vi "Grid Measurements Example - Topo & GridSpectr_DriftCorrection.vi"(6 "Internal use":string, 7 "Grid param":T1 {"height (m)" format="%#_6p"; "width (m)" format="%#_6p"; "center Y (m)" format="%#_6p"; "center X (m)" format="%#_6p"}, 8 "Error in (no error)":errorcluster, 9 "Points Y/Index Y":i32, 10 "Points X/Index X":i32, 11 "Method":enum16{"init", "run", "end"}(ring)=enum."end") -> (0 "Error out":errorcluster)   [LabVIEW 2014]
doc: "Example of a measurement VI to be used in the \"Experiments on a Grid\" tool as external VI.\n\nThis example measure the topography and spectroscopy data. The spectroscopy measurements are taken on a subgrid. The data are saved to a sxm and a binary file.\n\n- Nanonis Programming Interface -"
uses:
  <vilib>/Analysis/2dsp.llb/2D Cross Correlation (DBL).vi
  <userlib>/Nanonis Prog Interface V5/Nanonis Prog Interface.lvlib
  <vilib>/Analysis/NI_AALPro.lvlib
panel:
  in  "File name":string
  in  "STS Current":dbl format="%#_6p"
  in  "Imaging Current":dbl format="%#_6p"
  in  "zdrift \nDuration (s)":dbl
  in  "Correct z drift":bool
  out "Status":string="init"
  in  "Drift correction Pixels":i32=128 caption="Pixels for drift correction"
  out "Y Offset":dbl
  out "X Offset":dbl
  out "Points taken":dbl=1.0
  in  "Drift Correction":i32=128
  in  "Y subgrid spacing":u16=1
  in  "X subgrid spacing":u16=1
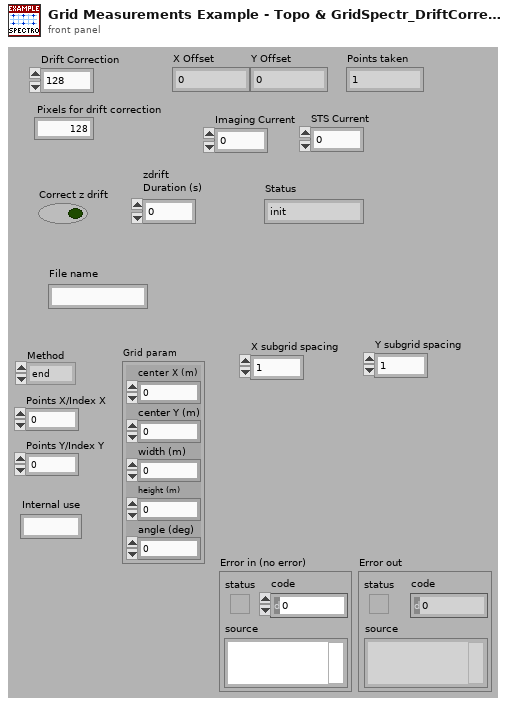
[diagram p1: front panel]
types:
  T1 = cluster{"center X (m)":sgl, "center Y (m)":sgl, "width (m)":sgl, "height (m)":sgl, "angle (deg)":sgl}
  T2 = enum16{"open", "replace", "create", "open or create", "replace or create", "replace or create with confirmation"}
  T3 = cluster{"center X":sgl, "center Y":sgl, "angle":sgl, "width":sgl, "height":sgl, "# pixels":i32, "# lines":i32}
  T4 = cluster{"Name":string, "Calibration":sgl, "Offset":sgl, "Channel index":i32}[]
  T5 = cluster{"up/down":bool, "time/line":sgl, "start time":timestamp, "end time":timestamp}
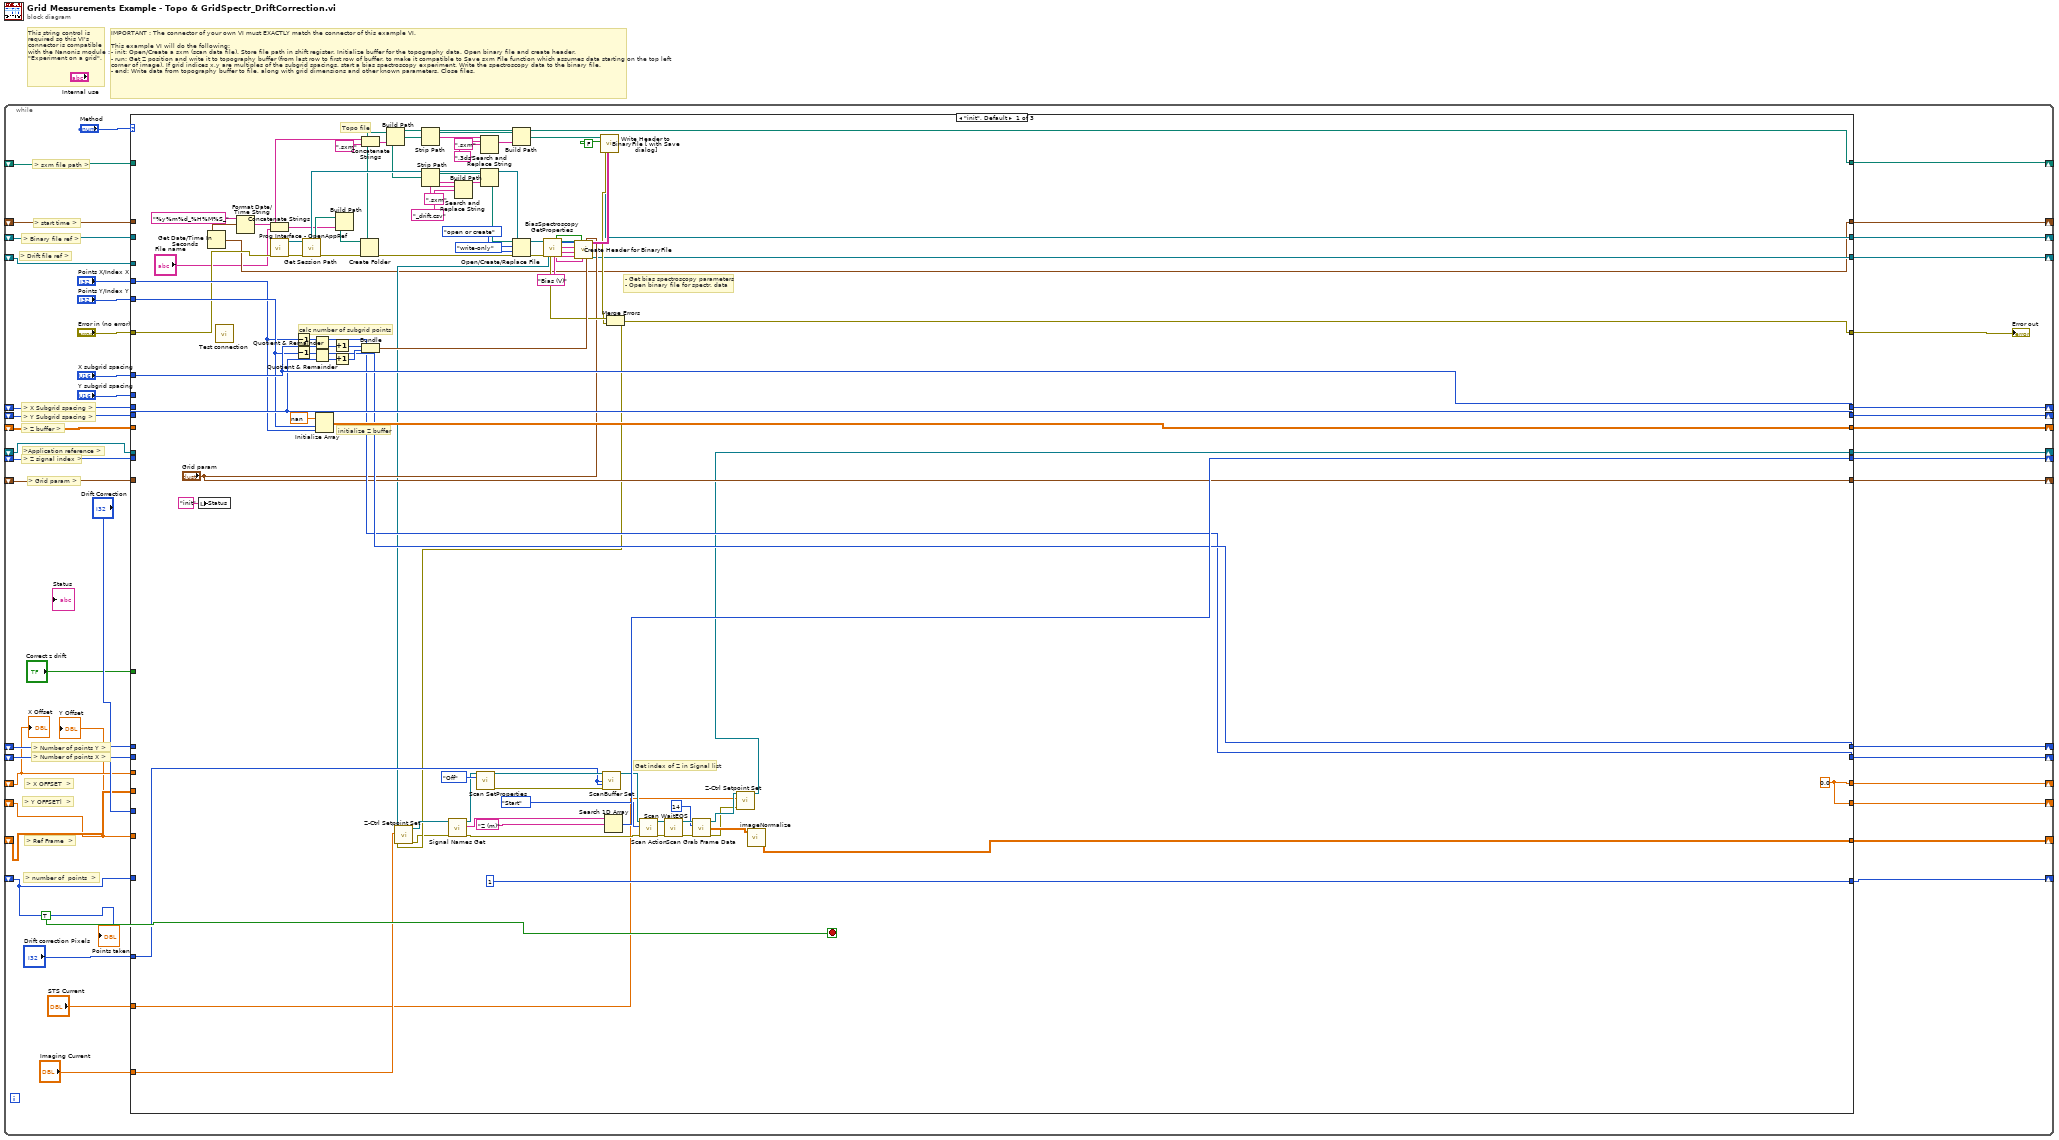
[diagram p0: block diagram]
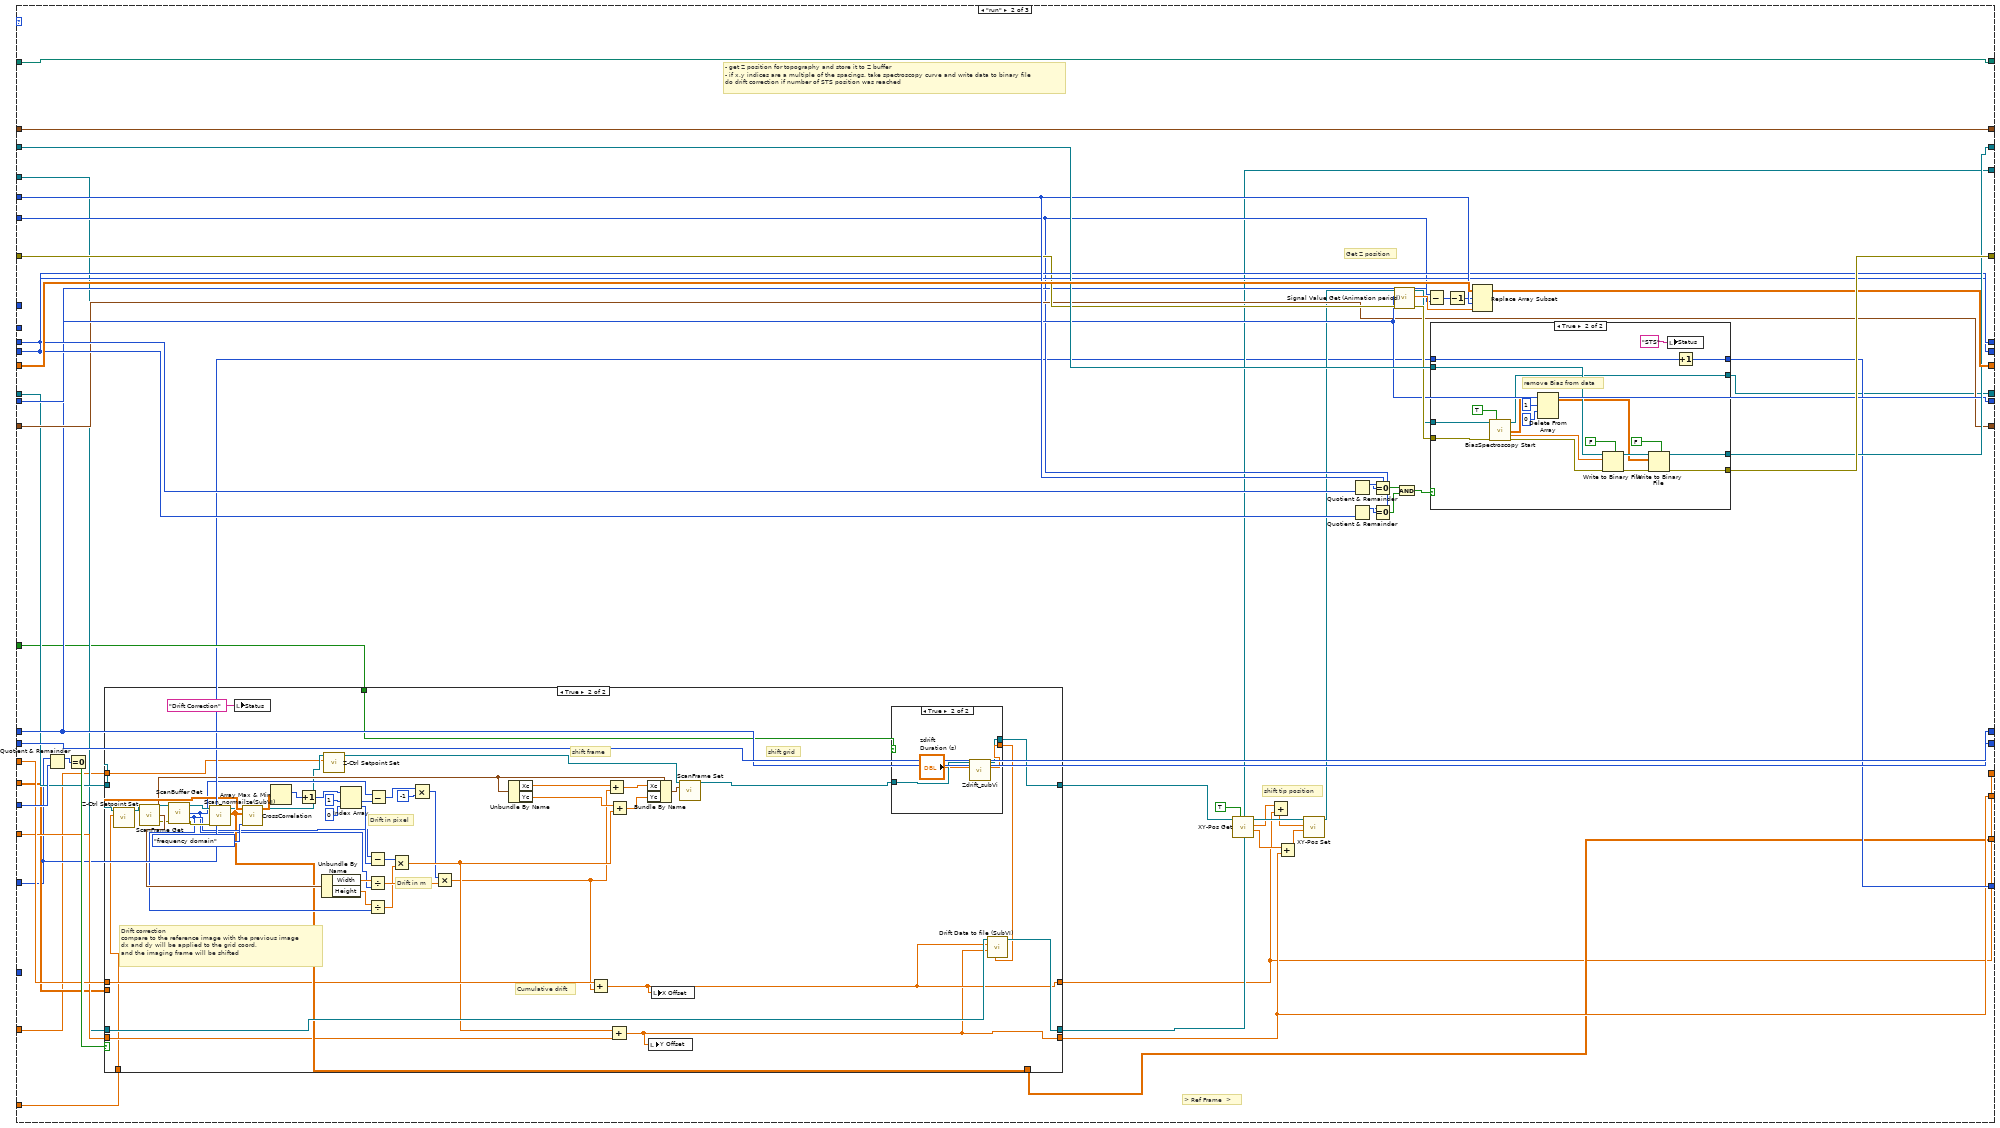
[diagram p2: hidden frame]
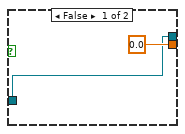
[diagram p4: hidden frame]
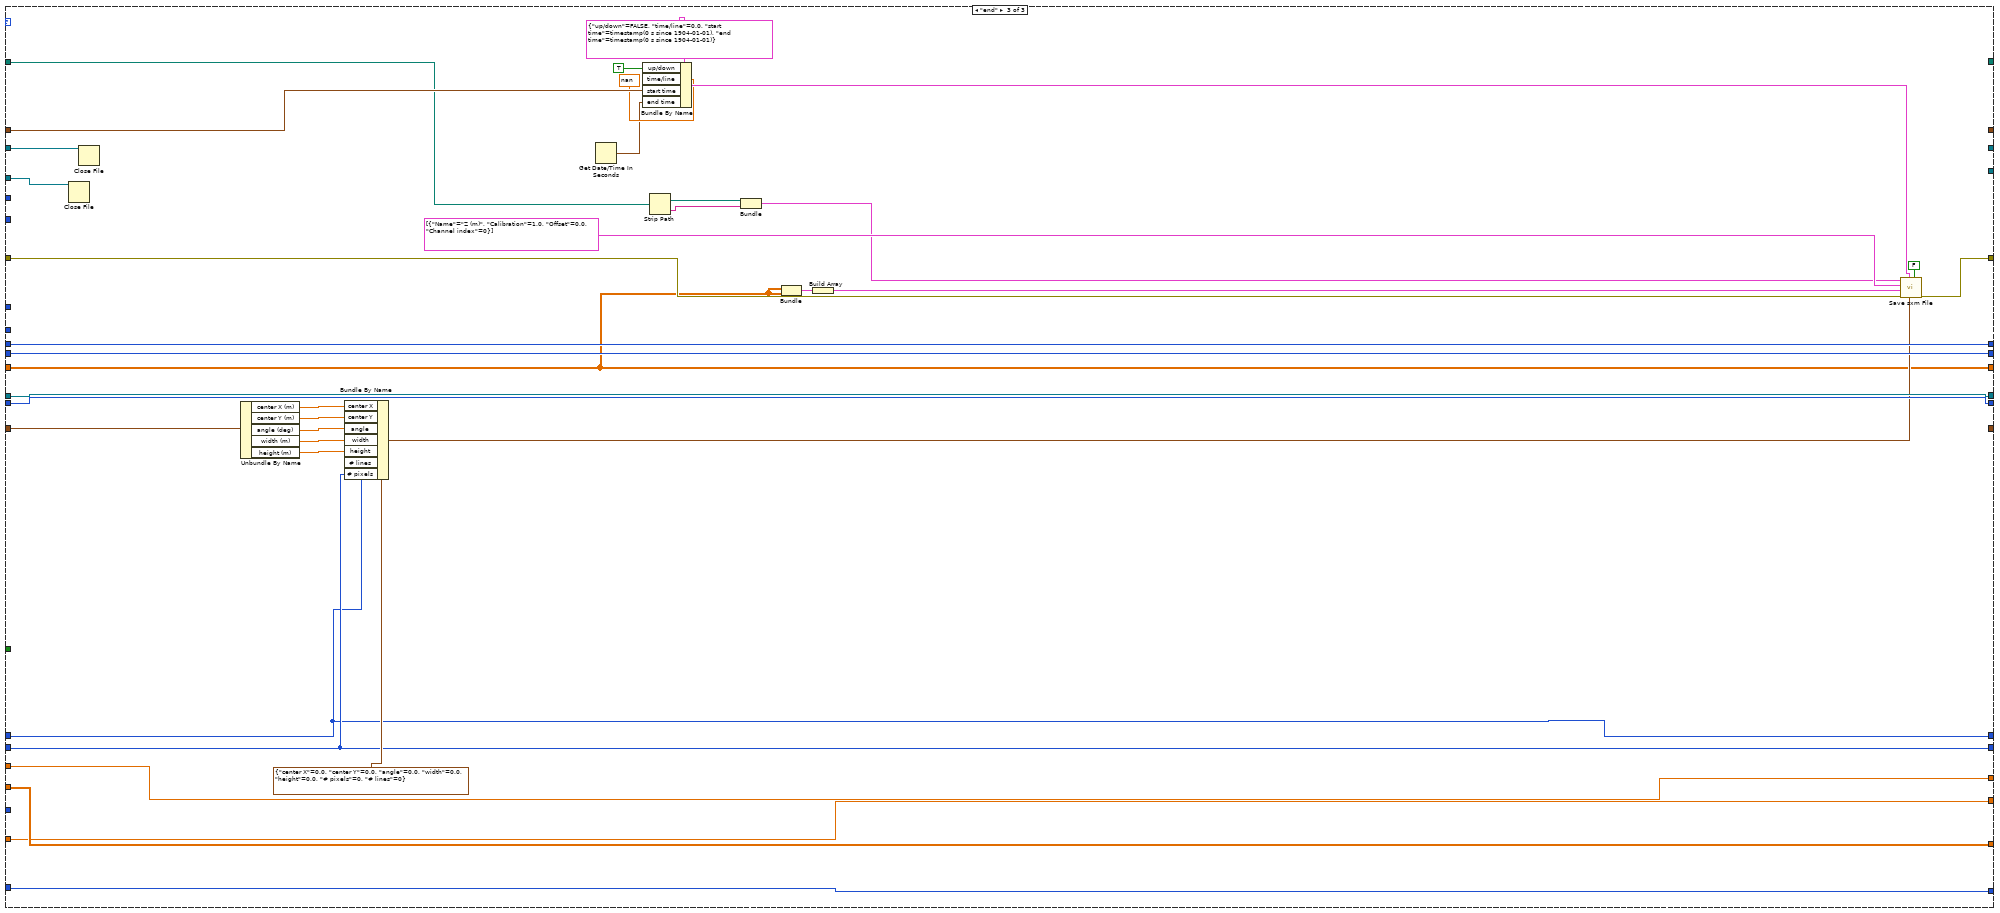
[diagram p6: hidden frame]
diagram:
  # "This string control is required so this VI's connector is compatible with the Nanonis module : \"Experiment on a grid\"."
  # "IMPORTANT : The connector of your own VI must EXACTLY match the connector of this example VI.\n\nThis example VI will do the following:\n- init: Open/Create a sxm (scan data file). Store file path in shift register. Initialize buffer for the topography data. Open binary file and create header.\n- run: Get Z position and write it to topography buffer (from last row to first row of buffer, to make it compatible to Save sxm File function which assumes data starting on the top left corner of image). If grid indices x,y are multiples of the subgrid spacings, start a bias spectroscopy experiment. Write the spectroscopy data to the binary file.\n- end: Write data from topography buffer to file, along with grid dimensions and other known parameters. Close files."
  n1 = while {
    shift-right: [w20] -> _
    shift-left: _ -> [w43]
    shift-right: [w38] -> _
    shift-left: _ -> [w37]
    shift-right: [w35] -> _
    shift-left: _ -> [w36]
    shift-right: [w34] -> _
    shift-left: _ -> [w33]
    shift-right: [w27] -> _
    shift-left: _ -> [w29]
    shift-right: [w28] -> _
    shift-left: _ -> [w30]
    shift-right: [w26] -> _
    shift-left: _ -> [w25]
    shift-right: [w24] -> _
    shift-left: _ -> [w23]
    shift-right: [w22] -> _
    shift-left: _ -> [w21]
    shift-right: [w19] -> _
    shift-left: _ -> [w18]
    shift-right: [w17] -> _
    shift-left: _ -> [w16]
    shift-right: [w15] -> _
    shift-left: _ -> [w8]
    shift-right: [w14] -> _
    shift-left: _ -> [w7]
    shift-right: [w13] -> _
    shift-left: _ -> [w10]
    shift-right: [w12] -> _
    shift-left: _ -> [w9]
    shift-right: [w5] -> _
    shift-left: _ -> [w4]
    stop <- TRUE stop-if-true
    # "> Drift file ref >"
    # "> number of  points  >"
    # "> Ref Frame  >"
    # "> Y OFFSETl  >"
    # "> X OFFSET  >"
    # "> Number of points X >"
    # "> Number of points Y >"
    # "> Grid param >"
    # "> start time >"
    # ">Application reference >"
    # "> Y Subgrid spacing >"
    # "> X Subgrid spacing >"
    # "> Z signal index >"
    # "> Binary file ref >"
    # "> Z buffer >"
    # "> sxm file path >"
    n2 = case shown="\"init\", Default" "Method" {
      tunnel: [w52 w185 _] -> w20
      tunnel: w43 -> [_ w185 w297]
      tunnel: "Error in (no error)" -> [w59 w171 w290]
      tunnel: [w69 w184 w289] -> w41
      tunnel: "Points X/Index X" -> [w108 w179 _]
      tunnel: "Points Y/Index Y" -> [w109 w163 _]
      tunnel: [w133 w182 w278] -> w38
      tunnel: w37 -> [_ w183 w278]
      tunnel: w36 -> [_ w181 w306]
      tunnel: [w124 w180 _] -> w35
      tunnel: [w122 w169 w307] -> w34
      tunnel: w33 -> [_ w169 w307]
      tunnel: "X subgrid spacing" -> [w121 _ _]
      tunnel: "Y subgrid spacing" -> [w120 _ _]
      tunnel: w30 -> [_ w173 w305]
      tunnel: w29 -> [_ w172 w304]
      tunnel: [w121 w173 w305] -> w28
      tunnel: [w120 w172 w304] -> w27
      tunnel: [w66 w154 w303] -> w26
      tunnel: w25 -> [_ w153 w303]
      tunnel: ["Grid param" w166 _] -> w24
      tunnel: w23 -> [_ w166 w288]
      tunnel: [w49 w167 _] -> w22
      tunnel: w21 -> [_ w167 w298]
      tunnel: [w109 w164 w279] -> w19
      tunnel: w18 -> [_ w164 w279]
      tunnel: [w108 w165 w280] -> w17
      tunnel: w16 -> [_ w165 w280]
      tunnel: [w98 w136 w277] -> w15
      tunnel: [w98 w143 w274] -> w14
      tunnel: [w74 w141 w276] -> w13
      tunnel: [1 w160 w275] -> w12
      tunnel: w9 -> [_ w137 w275]
      tunnel: "Drift Correction" -> [_ w158 _]
      tunnel: w10 -> [_ w142 w276]
      tunnel: w8 -> [_ w156 w277]
      tunnel: w7 -> [_ w155 w274]
      tunnel: "Drift correction Pixels" -> [w94 _ _]
      tunnel: [w87 w139 _] -> w5
      tunnel: w4 -> [_ w140 w271]
      tunnel: "Correct z drift" -> [_ w138 _]
      tunnel: "Imaging Current" -> [w70 w135 _]
      tunnel: "STS Current" -> [w64 w134 _]
      frame "init", Default {
        w98 = 0.0
        # "Topo file"
        # "- Get bias spectroscopy parameters\n- Open binary file for spectr. data"
        # "initialize Z buffer"
        # "calc number of subgrid points"
        # "Get index of Z in Signal list"
        n3 = local write "Status"("init" ("Status")) -> ()
        n4 = Get Date/Time In Seconds() -> (seconds since 1Jan1904=w49:timestamp)
        n5 = call <userlib>:"Test connection.vi"() -> ()  [unwired: 1 in]
        n6 = Format Date/Time String(time format string (%c)="%y%m%d_%H%M%S_", seconds (now)=w49) -> (date/time string=w48:string)  [unwired: 1 in]
        n7 = Concatenate Strings(w48, "File name") -> (w50:string)
        n8 = call <userlib>:"Prog Interface - OpenAppRef.vi"("Error in (no error)"=w59) -> ("Error out"=w61:errorcluster, "Application reference"=w63:refnum<vi>)  [unwired: 5 in]
        n9 = Decrement(x=w108) -> (x-1=w119:i32)
        n10 = Decrement(x=w109) -> (x-1=w118:i32)
        n11 = call <userlib>:"Get Session Path.vi"("error in (no error)"=w61, "Application ref in"=w63) -> ("error out"=w57:errorcluster, "Session path"=w60:path, "Application ref out"=w62:refnum<vi>)  [unwired: 7 in]
        n12 = Quotient & Remainder(x=w119, y=w121) -> (floor(x/y)=w117:i32)  [unwired: 1 out]
        n13 = Quotient & Remainder(x=w118, y=w120) -> (floor(x/y)=w116:i32)  [unwired: 1 out]
        n14 = Initialize Array(sgl nan ("element"), w109, w108) -> (w133:sgl[][])
        n15 = Increment(x=w117) -> (x+1=w115:i32)
        n16 = Increment(x=w116) -> (x+1=w114:i32)
        n17 = Build Path(base path=w60, name or relative path=w50) -> (appended path=w56:path)
        n18 = Create Folder(path (use dialog)=w56, error in=w57) -> (created path=w54:path, error out=w51:errorcluster)  [unwired: 1 in, 1 out]
        n19 = Concatenate Strings(w50, ".sxm" ("pattern")) -> (w53:string)
        n20 = Bundle(w115, w114) -> (w128:cluster{i32, i32})  [unwired: 1 in]
        n21 = Build Path(base path=w54, name or relative path=w53) -> (appended path=w52:path)
        n22 = Strip Path(path=w52) -> (stripped path=w80:path, name=w79:string)
        n23 = Strip Path(path=w52) -> (stripped path=w89:path, name=w85:string)
        n24 = Search and Replace String(input string=w85, search string=".sxm", replace string="_drift.csv" ("replace string (\"\")")) -> (result string=w86:string)  [unwired: 5 in, 3 out]
        n25 = Search and Replace String(input string=w79, search string=".sxm", replace string=".3ds" ("replace string (\"\")")) -> (result string=w81:string)  [unwired: 5 in, 3 out]
        n26 = Build Path(base path=w89, name or relative path=w86) -> (appended path=w88:path)
        n27 = Build Path(base path=w80, name or relative path=w81) -> (appended path=w76:path)
        n28 = Open/Create/Replace File(file path (use dialog)=w88, error in=w51, operation (0:open)=T2."open or create", access (0:read/write)=enum16{"read/write", "read-only", "write-only"}."write-only") -> (refnum out=w87:refnum<file>, error out=w58:errorcluster)  [unwired: 2 in, 1 out]
        n29 = call <userlib>:"BiasSpectroscopy GetProperties.vi"("Application ref in"=w62, "Error in (no error)"=w58) -> ("Backward sweep"=w129:bool, "Application ref out"=w72:refnum<vi>, "Number of points"=w111:i32, "Channels"=w110:string[], "Parameters"=w127:string[], "Fixed parameters"=w113:string[], "Error out"=w126:errorcluster)  [unwired: 5 in, 2 out]
        n30 = call <userlib>:"Create Header for BinaryFile.vi"("Grid points"=w128, "Grid param"="Grid param", "Fixed parameters"=w113, "Backward sweep"=w129, "Sweep signal"="Bias (V)" ("Sweep Signal"), "Parameters"=w127, "Channels"=w110, "Points per sweep"=w111) -> ("Header (fixed attributes)"=w131:string[][])  [unwired: 3 in]
        n31 = call <userlib>:"Write Header to BinaryFile [ with Save dialog].vi"("Fixed Attributes"=w131, "Show Dialog? (T)"=FALSE, "Filename"=w76) -> ("Error out"=w125:errorcluster, "File ref"=w124:refnum<file>)  [unwired: 5 in, 2 out]
        n32 = Merge Errors(w126, w125) -> (w69:errorcluster)
        n33 = call <userlib>:"Z-Ctrl Setpoint Set.vi"("error in (no error)"=w69, "Z Controller setpoint"=w70, "Application ref in"=w72) -> ("error out"=w68:errorcluster, "Application ref out"=w71:refnum<vi>)  [unwired: 7 in]
        n34 = call <userlib>:"Signal Names Get.vi"("error in (no error)"=w68, "Application ref in"=w71) -> ("error out"=w99:errorcluster, "Signals Names"=w112:string[], "Application ref out"=w93:refnum<vi>)  [unwired: 5 in]
        n35 = call <userlib>:"Scan SetProperties.vi"("Application ref in"=w93, "Continuous scan"=enum16{"No change", "On", "Off"}."Off") -> ("Application ref out"=w96:refnum<vi>, "Error out"=w95:errorcluster)  [unwired: 12 in]
        n36 = call <userlib>:"ScanBuffer Set.vi"("Application ref in"=w96, "Pixels"=w94, "Lines"=w94, "error in (no error)"=w95) -> ("Application ref out"=w92:refnum<vi>)  [unwired: 10 in, 1 out]
        n37 = Search 1D Array(1D array=w112, element="Z (m)") -> (index of element=w122:i32)  [unwired: 1 in]
        n38 = call <userlib>:"Scan Action.vi"("error in (no error)"=w99, "Scan action (Start)"=enum16{"Start", "Stop", "Pause", "Resume"}."Start", "Application ref in"=w92) -> ("error out"=w106:errorcluster, "Application ref out"=w105:refnum<vi>)  [unwired: 6 in]
        n39 = call <userlib>:"Scan WaitEOS.vi"("error in (no error)"=w106, "Application ref in"=w105) -> ("error out"=w103:errorcluster, "Application ref out"=w104:refnum<vi>)  [unwired: 5 in, 2 out]
        n40 = call <userlib>:"Scan Grab Frame Data.vi"("Application ref in"=w104, "Channel index (0-23)"=u8 14, "error in (no error)"=w103) -> ("Application ref out"=w67:refnum<vi>, "Scan frame data"=w73:sgl[][], "error out"=w65:errorcluster)  [unwired: 8 in, 2 out]
        n41 = call <userlib>:"Z-Ctrl Setpoint Set.vi"("error in (no error)"=w65, "Z Controller setpoint"=w64, "Application ref in"=w67) -> ("Application ref out"=w66:refnum<vi>)  [unwired: 7 in, 1 out]
        n42 = call "imageNormalize.vi"("Data"=w73) -> ("Array"=w74:dbl[][])  [unwired: 10 in]
      }
      frame "run" {
        # "> Ref Frame  >"
        # "shift tip position"
        # "Get Z position"
        # "- get Z position for topography and store it to Z buffer\n- if x,y indices are a multiple of the spacings, take spectroscopy curve and write data to binary file\ndo drift correction if number of STS position was reached"
        n43 = Quotient & Remainder(x=w137, y=w158) -> (x-y*floor(x/y)=w159:i32)  [unwired: 1 out]
        n44 = Equal To 0?(x=w159) -> (x = 0?=w157:bool)
        n45 = case shown="True" w157 {
          tunnel: w153 -> [w190 w201]
          tunnel: [w190 w212] -> w152
          tunnel: w142 -> [w187 w218]
          tunnel: [w189 w205] -> w136
          tunnel: [w188 w204] -> w143
          tunnel: w156 -> [w189 w209]
          tunnel: w155 -> [w188 w210]
          tunnel: [w187 w211] -> w141
          tunnel: w140 -> [w186 w217]
          tunnel: [w186 w216] -> w139
          tunnel: w138 -> [_ w208]
          tunnel: w135 -> [_ w199]
          tunnel: w134 -> [_ w196]
          frame False {
          }
          frame True {
            # "shift grid"
            # "Cumulative drift"
            # "shift frame"
            # "Drift in m"
            # "Drift in pixel"
            # "Drift correction \ncompare to the reference image with the previous image \ndx and dy will be applied to the grid coord, \nand the imaging frame will be shifted"
            n46 = call <userlib>:"Z-Ctrl Setpoint Set.vi"("Z Controller setpoint"=w199, "Application ref in"=w201) -> ("Application ref out"=w200:refnum<vi>)  [unwired: 8 in, 1 out]
            n47 = call <userlib>:"ScanFrame Get.vi"("Application ref in"=w200) -> ("Application ref out"=w234:refnum<vi>, "Center coordinates (m)"=w206:cluster{"Xc":sgl, "Yc":sgl}, "Size (m)"=w232:cluster{"Width":sgl, "Height":sgl}, "error out"=w231:errorcluster)  [unwired: 10 in, 1 out]
            n48 = call <userlib>:"ScanBuffer Get.vi"("Application ref in"=w234, "error in (no error)"=w231) -> ("Application ref out"=w230:refnum<vi>, "Pixels/line"=w207:i32, "Lines"=w220:i32, "error out"=w229:errorcluster)  [unwired: 9 in, 1 out]
            n49 = call "Scan_normailze(SubVI).vi"("error in (no error)"=w229, "Application in"=w230) -> ("Array"=w211:dbl[][], "Application out"=w198:refnum<vi>)  [unwired: 7 in, 1 out]
            n50 = local write "Status"("Drift Correction" ("Status")) -> ()
            n51 = call-poly <vilib>:"CrossCorrelation.vi"("algorithm"=enum32{"direct", "frequency domain"}."frequency domain", "Y"=w211, "X"=w218) -> ("Rxy"=w237:dbl[][])  [unwired: 7 in, 1 out]
            n52 = Array Max & Min(array=w237) -> (max index (indices)=w192:i32[])  [unwired: 3 out]
            n53 = Increment(x=w192) -> (x+1=w191:i32[])
            n54 = Unbundle By Name(w232) -> ("Width"=w228:sgl, "Height"=w233:sgl)
            n55 = call <userlib>:"Z-Ctrl Setpoint Set.vi"("Z Controller setpoint"=w196, "Application ref in"=w198) -> ("Application ref out"=w197:refnum<vi>)  [unwired: 8 in, 1 out]
            n56 = Index Array(array=w191, index #1=1 ("index"), index #2=0 ("index")) -> (element #1=w236:i32, element #2=w235:i32)
            n57 = Subtract(x=w220, y=w235) -> (x-y=w213:i32)
            n58 = Divide(x=w228, y=w207) -> (x/y=w227:sgl)
            n59 = Divide(x=w233, y=w220) -> (x/y=w226:sgl)
            n60 = Subtract(x=w207, y=w236) -> (x-y=w214:i32)
            n61 = Multiply(x=w213, y=w226) -> (x*y=w203:sgl)
            n62 = Multiply(x=w214, y=-1) -> (x*y=w194:i32)
            n63 = Multiply(x=w194, y=w227) -> (x*y=w202:sgl)
            n64 = Unbundle By Name(w206) -> ("Xc"=w224:sgl, "Yc"=w222:sgl)
            n65 = Add(x=w209, y=w202) -> (x+y=w205:dbl)
            n66 = Add(x=w224, y=w202) -> (x+y=w223:sgl)
            n67 = Add(x=w203, y=w210) -> (x+y=w204:dbl)
            n68 = Add(x=w222, y=w203) -> (x+y=w221:sgl)
            n69 = Bundle By Name(cluster=w206, "Xc"=w223, "Yc"=w221) -> (w225:cluster{"Xc":sgl, "Yc":sgl})
            n70 = local write "Y Offset"(w204) -> ()
            n71 = local write "X Offset"(w205) -> ()
            n72 = call <userlib>:"ScanFrame Set.vi"("Application ref in"=w197, "Center coordinates (m)"=w225) -> ("Application ref out"=w195:refnum<vi>)  [unwired: 12 in, 1 out]
            n73 = case shown="True" w208 {
              tunnel: [0.0 ("z drift") w246] -> w215
              tunnel: w195 -> [w241 w245]
              tunnel: [w241 w244] -> w212
              frame False {
              }
              frame True {
                n74 = call "Zdrift_subVi.vi"("Duration"="zdrift \nDuration (s)", "Application in"=w245) -> ("z drift"=w246:dbl, "Application out"=w244:refnum<vi>)  [unwired: 7 in, 1 out]
              }
            }
            n75 = call "Drift Data to file (SubVI).vi"("z drift"=w215, "y Drift"=w204, "X drift"=w205, "Byte Stream File in"=w217) -> ("Byte Stream File out"=w216:refnum<file>)  [unwired: 7 in]
          }
        }
        n76 = call <userlib>:"XY-Pos Get.vi"("Wait for newest data (F=False)"=TRUE, "Application ref in"=w152) -> ("Y (m)"=w147:sgl, "X (m)"=w148:sgl, "Application ref out"=w149:refnum<vi>)  [unwired: 5 in, 1 out]
        n77 = Add(x=w148, y=w136) -> (x+y=w146:dbl)
        n78 = Add(x=w147, y=w143) -> (x+y=w145:dbl)
        n79 = call <userlib>:"XY-Pos Set.vi"("Y (m)"=w145, "X (m)"=w146, "Application ref in"=w149) -> ("Application ref out"=w150:refnum<vi>)  [unwired: 5 in, 1 out]
        n80 = Quotient & Remainder(x=w179, y=w173) -> (x-y*floor(x/y)=w178:i32)  [unwired: 1 out]
        n81 = Quotient & Remainder(x=w163, y=w172) -> (x-y*floor(x/y)=w177:i32)  [unwired: 1 out]
        n82 = Equal To 0?(x=w178) -> (x = 0?=w176:bool)
        n83 = Equal To 0?(x=w177) -> (x = 0?=w175:bool)
        n84 = call <userlib>:"Signal Value Get (Animation period).vi"("error in (no error)"=w171, "Signal index (0-47)"=w169, "Application ref in"=w150) -> ("error out"=w170:errorcluster, "Signal value"=w168:sgl, "Application ref out"=w151:refnum<vi>)  [unwired: 5 in]
        n85 = And(x=w176, y=w175) -> (x .and. y?=w174:bool)
        n86 = Subtract(x=w164, y=w163) -> (x-y=w162:i32)
        n87 = case shown="True" w174 {
          tunnel: [w249 w254] -> w184
          tunnel: w181 -> [w250 w270]
          tunnel: [w250 w268] -> w180
          tunnel: w170 -> [w249 w267]
          tunnel: w151 -> [w248 w259]
          tunnel: [w248 w258] -> w154
          tunnel: [w247 w252] -> w160
          tunnel: w137 -> [w247 w253]
          frame False {
            # "Point indices aren't multiple of subgrid spacing\n=> no spectroscopy at this point"
          }
          frame True {
            # "remove Bias from data"
            n88 = call <userlib>:"BiasSpectroscopy Start.vi"("Application ref in"=w259, "Get data (F)"=TRUE ("Get Data (F)"), "Error in (no error)"=w267) -> ("Application ref out"=w258:refnum<vi>, "Data"=w266:sgl[][], "Parameters"=w265:sgl[], "Error out"=w256:errorcluster)  [unwired: 8 in, 1 out]
            n89 = Delete From Array(array=w266, length=1, index (row)=0 ("index")) -> (array with subset deleted=w264:sgl[][])  [unwired: 1 in, 1 out]
            n90 = Write to Binary File(file (use dialog)=w270, data=w265, error in=w256, 5:FALSE ("prepend array or string size? (T)")) -> (refnum out=w269:refnum<file>, error out=w255:errorcluster)  [unwired: 2 in, 1 out]
            n91 = Write to Binary File(file (use dialog)=w269, data=w264, error in=w255, 5:FALSE ("prepend array or string size? (T)")) -> (refnum out=w268:refnum<file>, error out=w254:errorcluster)  [unwired: 2 in, 1 out]
            n92 = local write "Status"("STS" ("Status")) -> ()
            n93 = Increment(x=w253) -> (x+1=w252:i32)
          }
        }
        n94 = Decrement(x=w162) -> (x-1=w161:i32)
        n95 = Replace Array Subset(array=w183, new element=w168, index (row)=w161, index (col)=w179) -> (w182:sgl[][])
      }
      frame "end" {
        n96 = Close File(refnum=w271) -> ()  [unwired: 1 in, 2 out]
        n97 = Close File(refnum=w306) -> ()  [unwired: 1 in, 2 out]
        n98 = Unbundle By Name(w288) -> ("center X (m)"=w286:sgl, "center Y (m)"=w285:sgl, "angle (deg)"=w284:sgl, "width (m)"=w283:sgl, "height (m)"=w282:sgl)
        n99 = Bundle By Name(cluster=T3 {"center X"=0.0, "center Y"=0.0, "angle"=0.0, "width"=0.0, "height"=0.0, "# pixels"=0, "# lines"=0} ("Scanfield"), "center X"=w286, "center Y"=w285, "angle"=w284, "width"=w283, "height"=w282, "# lines"=w279, "# pixels"=w280) -> (w281:T3)
        n100 = Get Date/Time In Seconds() -> (seconds since 1Jan1904=w273:timestamp)
        n101 = Bundle By Name(cluster=T5 {"up/down"=FALSE, "time/line"=0.0, "start time"=timestamp(0 s since 1904-01-01), "end time"=timestamp(0 s since 1904-01-01)} ("Scan param"), "up/down"=TRUE, "time/line"=sgl nan ("input 7"), "start time"=w298, "end time"=w273) -> (w296:T5)
        n102 = Strip Path(path=w297) -> (stripped path=w293:path, name=w292:string)
        n103 = Bundle("stripped path"=w293, "name"=w292) -> (w291:cluster{"stripped path":path, "name":string})  [unwired: 1 in]
        n104 = Bundle(w278, w278) -> (w302:cluster{sgl[][], sgl[][]})  [unwired: 1 in]
        n105 = Build Array(w302) -> (w301:cluster{sgl[][], sgl[][]}[])
        n106 = call <userlib>:"Save sxm File.vi"("Auto file naming? (T)"=FALSE, "Scanfield"=w281, "Scan param"=w296, "error in (no error)"=w290, "Channels data"=w301, "Channels config"=T4 [{"Name"="Z (m)", "Calibration"=1.0, "Offset"=0.0, "Channel index"=0}], "Filename control"=w291) -> ("error out"=w289:errorcluster)  [unwired: 2 in, 2 out]
      }
    }
    "Error out" <- w41
    "Points taken" <- w9
    "X Offset" <- w8
    "Y Offset" <- w7
  }
